vi "PhidgetGetDeviceID.vi"(0 "error in (no error)":errorcluster, 3 "Device In":u64) -> (7 "error out":errorcluster, 9 "Devie IDs":u32(ring) caption="Devie ID" items=["PHIDID_NOTHING", "PHIDID_INTERFACEKIT_4_8_8", "PHIDID_1000", "PHIDID_1001", "PHIDID_1002", "PHIDID_1008", "PHIDID_1010_1013_1018_1019", "PHIDID_1011", "PHIDID_1012", "PHIDID_1014", "PHIDID_1015", "PHIDID_1016", "PHIDID_1017", "PHIDID_1023", "PHIDID_1024", "PHIDID_1030", "PHIDID_1031", "PHIDID_1032", "PHIDID_1040", "PHIDID_1041", "PHIDID_1042", "PHIDID_1043", "PHIDID_1044", "PHIDID_1045", "PHIDID_1046", "PHIDID_1047", "PHIDID_1048", "PHIDID_1049", "PHIDID_1050", "PHIDID_1051", "PHIDID_1052", "PHIDID_1053", "PHIDID_1054", "PHIDID_1055", "PHIDID_1056", "PHIDID_1057", "PHIDID_1058", "PHIDID_1059", "PHIDID_1060", "PHIDID_1061", "PHIDID_1062", "PHIDID_1063", "PHIDID_1064", "PHIDID_1065", "PHIDID_1066", "PHIDID_1067", "PHIDID_1202_1203", "PHIDID_1204", "PHIDID_1215__1218", "PHIDID_1219__1222", "PHIDID_ADP1000", "PHIDID_DAQ1000", "PHIDID_DAQ1200", "PHIDID_DAQ1300", "PHIDID_DAQ1301", "PHIDID_DAQ1400", "PHIDID_DAQ1500", "PHIDID_DCC1000", "PHIDID_DST1000", "PHIDID_DST1200", "PHIDID_ENC1000", "PHIDID_HIN1000", "PHIDID_HIN1001", "PHIDID_HIN1100", "PHIDID_HUB0000", "", "", "PHIDID_HUB0004", "", "PHIDID_HUM1000", "PHIDID_LCD1100", "PHIDID_LED1000", "PHIDID_LUX1000", "PHIDID_MOT1100", "PHIDID_MOT1101", "PHIDID_OUT1000", "PHIDID_OUT1001", "PHIDID_OUT1002", "PHIDID_OUT1100", "PHIDID_PRE1000", "PHIDID_RCC1000", "PHIDID_REL1000", "PHIDID_REL1100", "PHIDID_REL1101", "PHIDID_SAF1000", "PHIDID_SND1000", "PHIDID_DCC1000", "PHIDID_STC1000", "PHIDID_TMP1000", "PHIDID_TMP1100", "PHIDID_TMP1101", "PHIDID_VCP1000", "PHIDID_VCP1001", "PHIDID_VCP1002", "PHIDID_DITITALINPUT_PORT", "PHIDID_DIGITALOUTPUT_PORT", "PHIDID_VOLTAGEINPUT_PORT", "PHIDID_VOLTAGERATIOINPUT_PORT", "", "", "", "", "", "", "", "PHIDID_VCP1100", "", "", "PHIDID_DCC1100", "PHIDID_HIN1101", "PHIDID_DCC1001", "PHIDID_DICTIONARY", "", "", "", "PHIDID_STC1001", "", "PHIDID_DCC1002", "PHIDID_STC1002", "PHIDID_STC1003", "PHIDID_DCC1003", "PHIDID_DST1001", "", "PHIDID_HUB5000", "PHIDID_RCC0004", "PHIDID_UNKNOWN", "", "PHIDID_HUM1001"], 10 "Device Out":u64)   [LabVIEW 2020, in "Phidget Common.lvlib"]
doc: "${DeviceID:Header}"
uses:
  <instrlib>/Phidgets/Phidget Common/Phidget Common.lvlib
  phidget22.dll
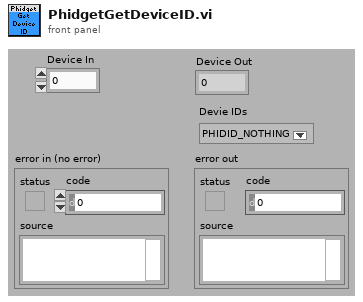
[diagram p1: front panel]
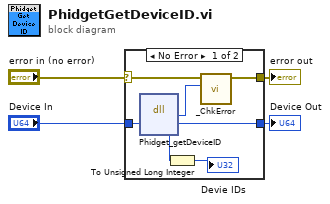
[diagram p0: block diagram]
diagram:
  n1 = case shown="No Error" "error in (no error)" {
    selector: "error in (no error)" -> [w11 w13]
    tunnel: [w10 w13] -> w3
    tunnel: "Device In" -> [w8 w12]
    tunnel: [w9 w12] -> w1
    frame No Error {
      n2 = dll-call lib="phidget22.dll" fn="Phidget_getDeviceID"("phid"=w8) -> ("return type"=w7:i32, "phid"=w9:u64, "DeviceID"=w5:i32)  [unwired: 4 in, 2 out]
      n3 = To Unsigned Long Integer(number=w5) -> (unsigned 32bit integer=→"Devie IDs":u32)
      n4 = call <instrlib>:"_ChkError.vi"("Return Code"=w7, "error in (no error)"=w11) -> ("error out"=w10:errorcluster)  [unwired: 9 in]
    }
    frame Error {
    }
  }
  "error out" <- w3
  "Device Out" <- w1
